vi "SRAM内存管理实验.vi"() -> ()   [LabVIEW 2011]
uses:
  <vilib>/STM32_DriverVI_Interface_F4/SRAM/SRAM Style_F4.ctl
  <vilib>/STM32_DriverVI_Interface_F4/SRAM/SRAM Write_F4.vi
panel:
  out "value":u8
  in  "Memory Free":bool
  out "SRAM Memory Usage（%）":u16
  out "SRAM_Size（KB）":u16
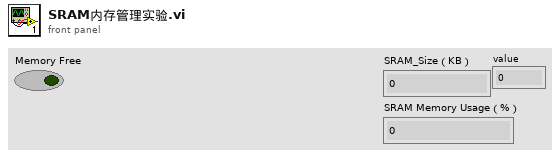
[diagram p1: front panel]
types:
  T1 = typedef "SRAM Style_F4.ctl" = enum8{"SRAM_Inner (24KB)", "SRAM_Extern (768KB)", "SRAM_CCM (48KB)"}
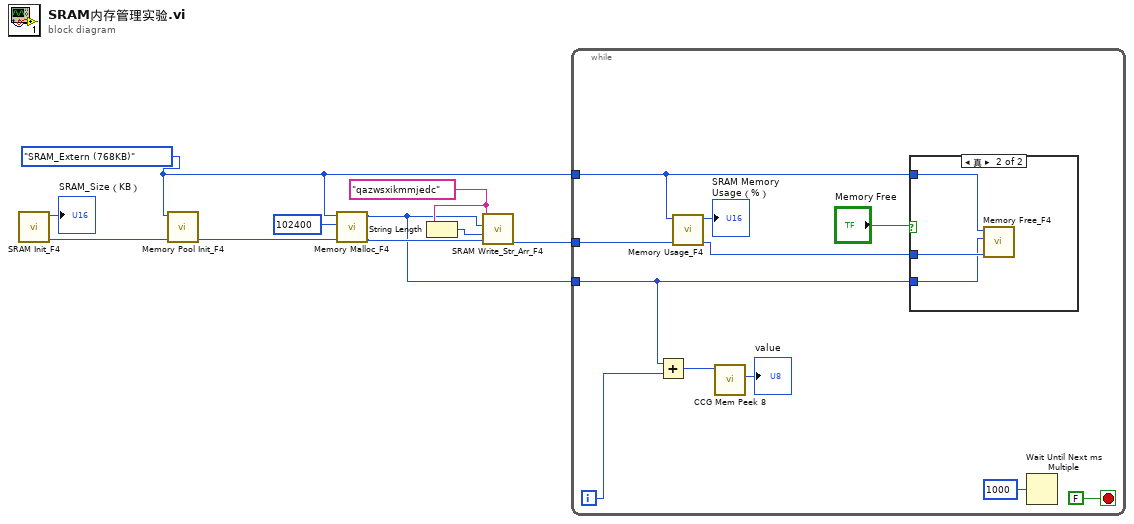
[diagram p0: block diagram]
diagram:
  w7 = "qazwsxikmmjedc" ("写入字符串")
  w1 = SRAM_Style_F4."SRAM_Extern (768KB)" ("SRAM Memory Zone")
  n1 = call <vilib>:"SRAM Init_F4.vi"() -> ("err_out"=w10:u8, "SRAM_Size（KB）"=→"SRAM_Size（KB）":u16)  [unwired: 10 in]
  n2 = call <vilib>:"Memory Pool Init_F4.vi"("err_in"=w10, "SRAM Memory Zone"=w1) -> ("err_out"=w4:u8)  [unwired: 9 in]
  n3 = call <vilib>:"Memory Malloc_F4.vi"("err_in"=w4, "Apply Memory Size"=u32 102400, "SRAM Memory Zone"=w1) -> ("err_out"=w3:u8, "Memory First Address"=w2:u32)  [unwired: 7 in]
  n4 = String Length(string=w7) -> (length=w8:i32)
  n5 = call-poly <vilib>:"SRAM Write_Str_Arr_F4.vi"("err_in"=w3, "写入字节数"=w8, "写入起始地址（绝对地址）"=w2, "写入字符串"=w7) -> ("err_out"=w6:u8)  [unwired: 7 in]
  n6 = while {
    tunnel: w6 -> [w21]
    tunnel: w1 -> [w17]
    tunnel: w2 -> [w14]
    i -> [w13]
    stop <- FALSE stop-if-true
    n7 = Add(x=w14, y=w13) -> (x+y=w12:u32)
    n8 = call <vilib>:"Memory Usage_F4.vi"("err_in"=w21, "SRAM Memory Zone"=w17) -> ("err_out"=w20:u8, "SRAM Memory Usage（%）"=→"SRAM Memory Usage（%）":u16)  [unwired: 8 in]
    n9 = call <vilib>:"CCG Mem Peek 8.vi"("address in"=w12) -> ("value"=→"value":u8)  [unwired: 8 in, 2 out]
    n10 = case shown="真" "Memory Free" {
      tunnel: w20 -> [_ w24]
      tunnel: w17 -> [_ w23]
      tunnel: w14 -> [_ w22]
      frame False {
      }
      frame True {
        n11 = call <vilib>:"Memory Free_F4.vi"("err_in"=w24, "Memory First Address"=w22, "SRAM Memory Zone"=w23) -> ()  [unwired: 8 in, 1 out]
      }
    }
    n12 = Wait Until Next ms Multiple(millisecond multiple=u32 1000 ("毫秒倍数")) -> ()  [unwired: 1 out]
  }
